vi "Forward Auto Veer V.5.0.vi"() -> (2 "Right":dbl format="%#_13g", 3 "Left":dbl format="%#_13g")   [LabVIEW 2016]
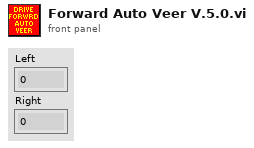
[diagram p1: front panel]
types:
  T1 = typedef "WPI_GyroDevRef.ctl" = cluster{"DevStatus":errorcluster, "Analog Channel":T2, "Offset":dbl, "Gain (VoltsPerDegree/Second)":dbl, "Gyro Type":enum16{"Analog", "XRS450"}, "Handle":i32, "SPI Bus":T3, "Device Found":bool, "Sample Rate":dbl, "Calibrate On Open":bool}
  T2 = typedef "FPGA_AIChannel.ctl" = enum8{"AI 0", "AI 1", "AI 2", "AI 3", "AI MXP 0", "AI MXP 1", "AI MXP 2", "AI MXP 3", "Invalid"}
  T3 = typedef "spi_bus.ctl" = enum16{"SPI On-Board, CS0", "SPI On-Board, CS1", "SPI On-Board, CS2", "SPI On-Board, CS3", "SPI MXP", "Invalid"}
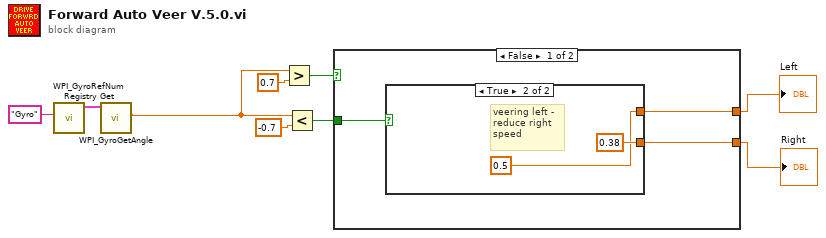
[diagram p0: block diagram]
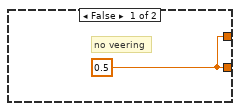
[diagram p2: hidden frame]
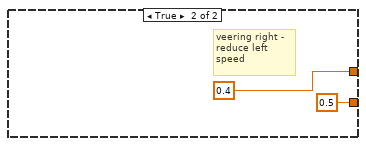
[diagram p3: hidden frame]
diagram:
  n1 = call <vilib>:"WPI_GyroRefNum Registry Get.vi"("refnum name"="Gyro") -> ("GyroDevRef"=w4:T1)  [unwired: 9 in, 1 out]
  n2 = call <vilib>:"WPI_GyroGetAngle.vi"("GyroDevRef"=w4) -> ("Angle"=w3:dbl)  [unwired: 6 in, 4 out]
  n3 = Greater?(x=w3, y=0.7) -> (0:w8:bool)
  n4 = Less?(x=w3, y=-0.7) -> (x < y?=w6:bool)
  n5 = case shown="False" w8 {
    tunnel: w6 -> [w12 _]
    tunnel: [w11 0.5] -> w2
    tunnel: [w10 0.4] -> w1
    frame False {
      n6 = case shown="True" w12 {
        tunnel: [w13 0.38] -> w11
        tunnel: [w13 0.5] -> w10
        frame False {
          w13 = 0.5
          # "no veering"
        }
        frame True {
          # "veering left - \nreduce right\nspeed"
        }
      }
    }
    frame True {
      # "veering right - \nreduce left \nspeed"
    }
  }
  "Left" <- w1
  "Right" <- w2
